vi "Default Path.vi"() -> (0 "base path":path)   [LabVIEW 2019, in "FP-TC-Shared.lvclass"]
uses:
  FP-TC-Shared.lvclass
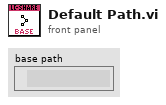
[diagram p1: front panel]
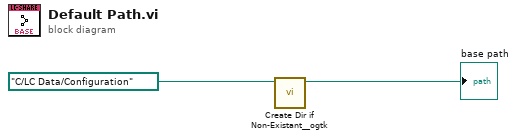
[diagram p0: block diagram]
diagram:
  n1 = call <userlib>:"Create Dir if Non-Existant__ogtk.vi"("Directory Path"=path "C:/LC Data/Configuration" ("Relative path (.)")) -> ("dup Directory Path"=→"base path":path)  [unwired: 8 in, 2 out]
